vi "HAPS_PhaseGainSweep_Preamp_Chs.vi"() -> ()   [LabVIEW 2023, in "HAPS.lvlib"]
uses:
  HAPS.lvlib
  HAPS_SerialPort.ctl
  MCU_Function.ctl
  set_ele.ctl
  HAPS_MCU_ELE_Func.ctl
  R_S/R_S.lvlib
panel:
  in  "Init?":bool=TRUE
  in  "Gain sweep res":i32=3
  in  "Gain_Start":i32
  in  "Phase Sweep Step":i32=64
  in  "Gain Sweep Step":i32=13
  in  "comn_gain":i32=17
  out "Each_Phase_Sweep(sec)":dbl
  out "dup path":path
  out "Gain_step":i32
  out "channel":i32
  out "chain_id":i32
  out "group":i32
  out "array_id":i32
  in  "File_note":string
  out "Duration(sec)":dbl
  out "In-Phase : Phase(degree)":dbl[](graph)
  out "In-Phase : Gain(dB)":dbl[](graph)
  in  "Tx/Rx":enum16{"Rx", "Tx"}(ring)=enum."Tx"
  in  "array_id (MCU index)":i32
  in  "MCU_UART_addr":refnum<visa-resource-name>="COM8"
  in  "Target(degree)":dbl format="%#_13g"
  in  "SweepPoints":i32=11
  in  "sParameter":i32=21
  in  "Stop_Freq(GHz)":dbl=39.5
  in  "Start_Freq(GHz)":dbl=38.5
  in  "VISA resource name":refnum<visa-resource-name>="TCPIP0::192.168.119.45::inst0::INSTR"
  in  "HAPS_Equipment":enum16{"Keysight", "R&S"}(ring)=enum."R&S"
  # "HAPS_24x24_PhaseGain_Sweep_Preamp_v1.8"
  # "K:4718\nR:2798"
  # "VNA"
  # "Test Status"
  # "DUT"
  # "TCPIP0::192.168.1.31::hislip0::INSTR"
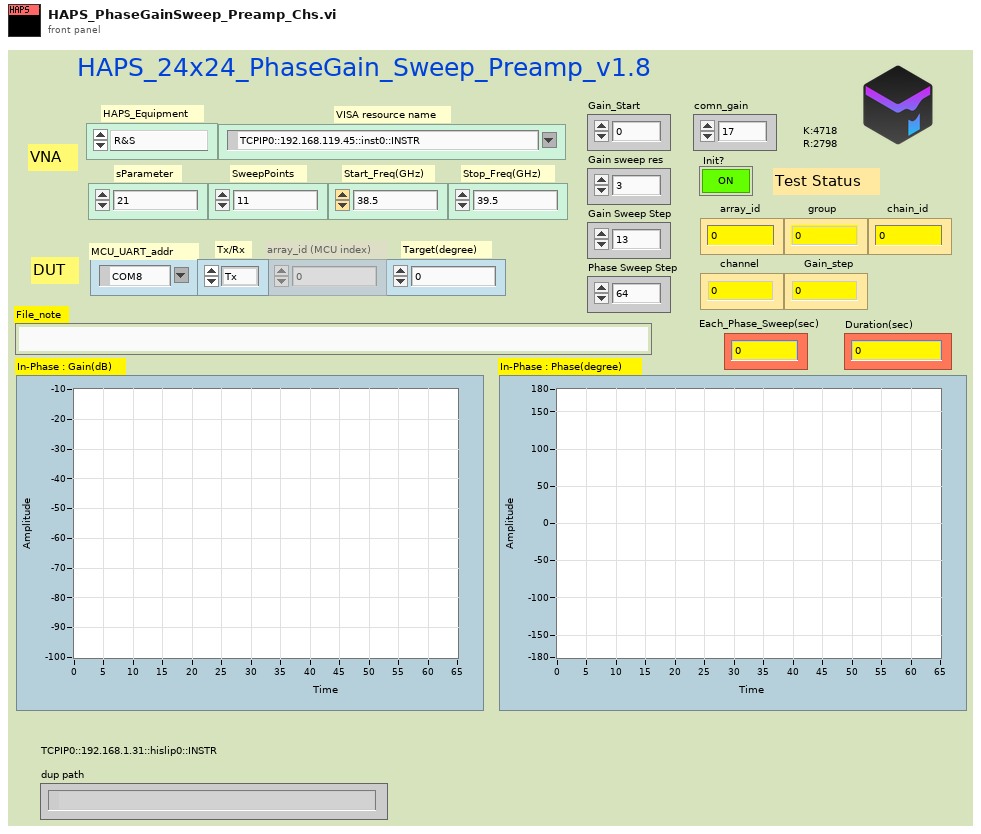
[diagram p1: front panel]
types:
  T1 = typedef "HAPS.lvlib/HAPS_SerialPort.ctl" = enum16{"Init", "Close", "CMD", "Flush"}
  T2 = typedef "HAPS.lvlib/HAPS_MCU_ELE_Func.ctl" = enum16{"array_init", "set_com_gain", "set_ch_gain_phase", "set_pd_range", "get_preamp_temp", "get_bfic_temp", "get_tx_pd", "ch_on", "ch_on_2", "ch_ctrl_all", "array_ctrl_src"}
  T3 = typedef "HAPS.lvlib/MCU_Function.ctl" = cluster{"Tx/Rx":enum16{"Rx", "Tx"}, "Enable?":enum16{"OFF", "On"}, "Source":enum16{"MCU", "ACU"}}
  T4 = typedef "HAPS.lvlib/set_ele.ctl" = cluster{"ch":i32, "chain_id":i32, "group":i32, "array_id":i32, "ele_phase":i32, "ele_gain":i32, "com_gain":i32, "pd_range":i32}
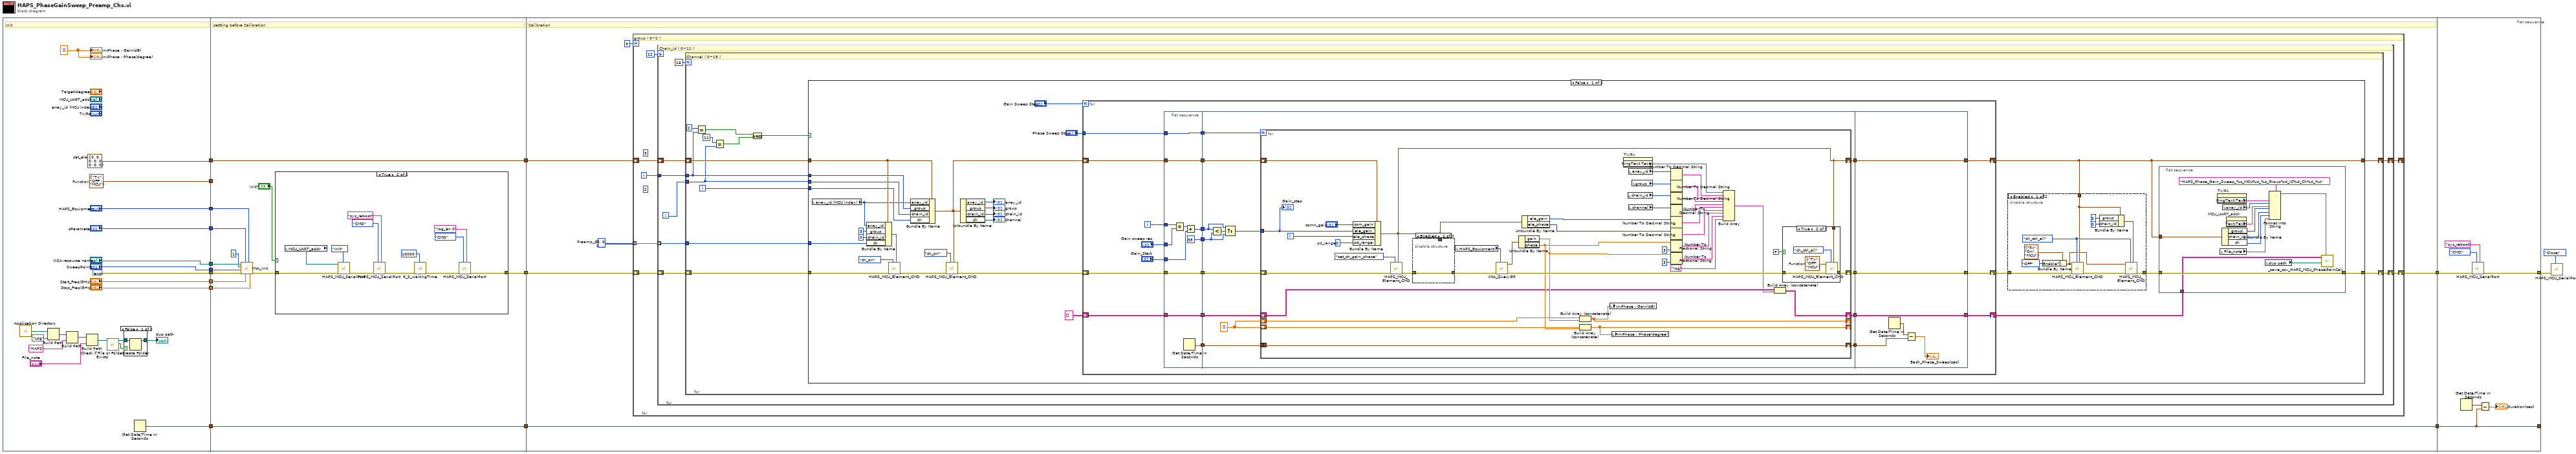
[diagram p0: block diagram]
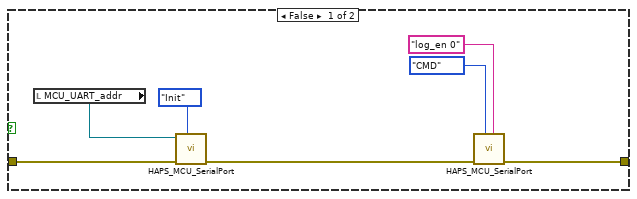
[diagram p3: hidden frame]
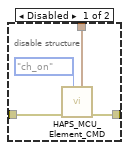
[diagram p4: hidden frame]
diagram:
  n1 = flat-sequence {
    tunnel: [w31] -> w17
    tunnel: [w38] -> w16
    tunnel: [errorcluster {"status"=FALSE, "code"=0, "source"=""} ("error in")] -> w14
    tunnel: ["sParameter"] -> w12
    tunnel: ["VISA resource name"] -> w11
    tunnel: ["Start_Freq(GHz)"] -> w10
    tunnel: ["Stop_Freq(GHz)"] -> w9
    tunnel: ["SweepPoints"] -> w8
    tunnel: ["HAPS_Equipment"] -> w7
    tunnel: [w28] -> w5
    tunnel: w17 -> [w54]
    tunnel: w16 -> [_]
    tunnel: [w54] -> w15
    tunnel: w14 -> [w53]
    tunnel: [w45] -> w13
    tunnel: w12 -> [w52]
    tunnel: w11 -> [w51]
    tunnel: w10 -> [w50]
    tunnel: w9 -> [w49]
    tunnel: w8 -> [w48]
    tunnel: w7 -> [w44]
    tunnel: [w43] -> w6
    tunnel: w5 -> [w43]
    tunnel: w15 -> [w78]
    tunnel: w13 -> [w79]
    tunnel: w6 -> [w76]
    tunnel: [w76] -> w4
    tunnel: [w74] -> w3
    tunnel: [w273] -> _
    tunnel: w4 -> [w273]
    tunnel: w3 -> [w269]
    tunnel: [w268] -> w2
    frame #0 {
      w29 = dbl[] []
      w31 = T4 {"ch"=0, "chain_id"=0, "group"=0, "array_id"=0, "ele_phase"=0, "ele_gain"=0, "com_gain"=0, "pd_range"=0}  # set_ele
      w38 = T3 {"Tx/Rx"=enum."Tx", "Enable?"=enum."OFF", "Source"=enum."MCU"}  # Function
      # "Init"
      n2 = call <vilib>:"Application Directory.vi"() -> ("Application Directory"=w26:path)
      n3 = Build Path(base path=w26, name or relative path="Log") -> (appended path=w27:path)
      n4 = Build Path(base path=w27, name or relative path="HAPS") -> (appended path=w23:path)
      n5 = Build Path(base path=w23, name or relative path="File_note") -> (appended path=w21:path)
      n6 = call <vilib>:"Check if File or Folder Exists.vi"("path"=w21) -> ("file or folder exists?"=w20:bool, "dup path"=w19:path)  [unwired: 8 in, 1 out]
      n7 = case shown="False" w20 {
        tunnel: w19 -> [w40 w41]
        tunnel: [w39 w41] -> w18
        frame False {
          n8 = Create Folder(path (use dialog)=w40) -> (created path=w39:path)  [unwired: 2 in, 2 out]
        }
        frame True {
        }
      }
      "dup path" <- w18
      n9 = Get Date/Time In Seconds() -> (seconds since 1Jan1904=w28:timestamp)
      "In-Phase : Gain(dB)" <- w29
      "In-Phase : Phase(degree)" <- w29
    }
    frame #1 {
      # "settting before Calibration"
      n10 = call "VNA_init.vi"("Stop_Freq(GHz)"=w49, "HAPS_MCU_CMD"=w44, "Start_Freq(GHz)"=w50, "sParameter"=w52, "error in"=w53, "SweepPoints"=w48, "Mark no."=1, "VISA resource name"=w51) -> ("error out"=w46:errorcluster)  [unwired: 3 in]
      n11 = case shown="True" "Init?" {
        tunnel: w46 -> [w58 w71]
        tunnel: [w55 w68] -> w45
        frame False {
          n12 = local read "MCU_UART_addr"() -> (w56:refnum<visa-resource-name>)
          n13 = call "HAPS_MCU_SerialPort.vi"("HAPS_SerialPort_Func"=HAPS_SerialPort."Init", "error in"=w58, "VISA resource name"=w56) -> ("error out"=w59:errorcluster)  [unwired: 6 in, 2 out]
          n14 = call "HAPS_MCU_SerialPort.vi"("Command"="log_en 0", "HAPS_SerialPort_Func"=enum16{"Init", "Close", "CMD"}."CMD" ("HAPS_SerialPort"), "error in"=w59) -> ("error out"=w55:errorcluster)  [unwired: 6 in, 2 out]
        }
        frame True {
          n15 = local read "MCU_UART_addr"() -> (w69:refnum<visa-resource-name>)
          n16 = call "HAPS_MCU_SerialPort.vi"("HAPS_SerialPort_Func"=HAPS_SerialPort."Init", "error in"=w71, "VISA resource name"=w69) -> ("error out"=w65:errorcluster)  [unwired: 6 in, 2 out]
          n17 = call "HAPS_MCU_SerialPort.vi"("Command"="sys_reboot", "HAPS_SerialPort_Func"=enum16{"Init", "Close", "CMD"}."CMD" ("HAPS_SerialPort"), "error in"=w65) -> ("error out"=w64:errorcluster)  [unwired: 6 in, 2 out]
          n18 = call "R_S_waitingTime.vi"("Waiting Time(ms)"=u32 10000, "error in"=w64) -> ("error out"=w63:errorcluster)  [unwired: 9 in]
          n19 = call "HAPS_MCU_SerialPort.vi"("Command"="log_en 0", "HAPS_SerialPort_Func"=enum16{"Init", "Close", "CMD"}."CMD" ("HAPS_SerialPort"), "error in"=w63) -> ("error out"=w68:errorcluster)  [unwired: 6 in, 2 out]
        }
      }
    }
    frame #2 {
      w75 = i32[][] [[2, 0, 0, 8, 8, 10, 11, 9, 9, 1, 1, 3], [3, 1, 1, 9, 9, 11, 13, 15, 15, 7, 7, 5], [5, 7, 7, 15, 15, 13, 14, 14, 6, 6, 4, 12]]  # Preamp_ch
      # "Calibration"
      n20 = for {
        N: 3 -> [_]
        shift-right: [w80] -> _
        shift-left: w78 -> [w84]
        shift-right: [w86] -> w74
        shift-left: w79 -> [w85]
        tunnel: w75 -> [w81] mode=indexing
        i -> [w82]
        (unwired) 2
        (unwired) 3
        # "group ( 0~2 )"
        n21 = for {
          N: 12 -> [_]
          shift-right: [w88] -> w80
          shift-left: w84 -> [w92]
          shift-right: [w87] -> w86
          shift-left: w85 -> [w93]
          tunnel: w82 -> [w91]
          tunnel: w81 -> [w89] mode=indexing
          i -> [w90]
          # "Chain_id ( 0~11 )"
          n22 = for {
            N: 16 -> [_]
            shift-right: [w104] -> w88
            shift-left: w92 -> [w107]
            shift-right: [w105] -> w87
            shift-left: w93 -> [w106]
            tunnel: w91 -> [w103]
            tunnel: w90 -> [w96]
            tunnel: w89 -> [w95]
            i -> [w97]
            # "Channel ( 0~15 )"
            n23 = Equal?(x=2, y=w103) -> (x = y?=w100:bool)
            n24 = Equal?(x=11, y=w96) -> (x = y?=w99:bool)
            n25 = And(x=w100, y=w99) -> (x .and. y?=w98:bool)
            n26 = case shown="False" w98 {
              tunnel: w107 -> [w125 w267]
              tunnel: w97 -> [w132 _]
              tunnel: w106 -> [w126 w266]
              tunnel: w103 -> [w134 _]
              tunnel: w96 -> [w133 _]
              tunnel: [w116 w266] -> w105
              tunnel: [w115 w267] -> w104
              tunnel: w95 -> [w120 _]
              frame False {
                n27 = local read "array_id (MCU index)"() -> (w123:i32)
                n28 = Bundle By Name(cluster=w125, "array_id"=w123, "group"=3, "chain_id"=0, "ch"=w120) -> (w124:T4)
                n29 = call "HAPS_MCU_Element_CMD.vi"("set_ele"=w124, "HAPS_MCU_ELE_Func."=HAPS_MCU_ELE_Func."ch_on", "error in"=w126) -> ("error out"=w127:errorcluster)  [unwired: 7 in, 1 out]
                n30 = Bundle By Name(cluster=w125, "array_id"=w123, "group"=w134, "chain_id"=w133, "ch"=w132) -> (w112:T4)
                n31 = call "HAPS_MCU_Element_CMD.vi"("set_ele"=w112, "HAPS_MCU_ELE_Func."=HAPS_MCU_ELE_Func."ch_on", "error in"=w127) -> ("error out"=w130:errorcluster)  [unwired: 7 in, 1 out]
                n32 = Unbundle By Name(w112) -> ("array_id"=→"array_id":i32, "group"=→"group":i32, "chain_id"=→"chain_id":i32, "ch"=→"channel":i32)
                n33 = for {
                  N: "Gain Sweep Step" -> [_]
                  shift-right: [w166] -> w129
                  shift-left: w130 -> [w167]
                  shift-right: [w165] -> w115
                  shift-left: w112 -> [w164]
                  shift-right: [w163] -> w114
                  shift-left: string[][] [] -> [w168]
                  tunnel: "Phase Sweep Step" -> [w152]
                  i -> [w162]
                  n34 = flat-sequence {
                    tunnel: w162 -> [w176]
                    tunnel: w164 -> [w177]
                    tunnel: w167 -> [w178]
                    tunnel: w168 -> [w179]
                    tunnel: [w179] -> w161
                    tunnel: [w178] -> w160
                    tunnel: [w177] -> w159
                    tunnel: [w175] -> w158
                    tunnel: [w174] -> w153
                    tunnel: w152 -> [w174]
                    tunnel: "Gain sweep res" -> [w173]
                    tunnel: "Gain_Start" -> [w171]
                    tunnel: [w170] -> w149
                    tunnel: [35 ("y")] -> w148
                    tunnel: w161 -> [w193]
                    tunnel: w160 -> [w192]
                    tunnel: w159 -> [w189]
                    tunnel: w158 -> [w186]
                    tunnel: [w191] -> w157
                    tunnel: [w190] -> w156
                    tunnel: [w188] -> w155
                    tunnel: [w185] -> w154
                    tunnel: w153 -> [w184]
                    tunnel: w149 -> [w182]
                    tunnel: w148 -> [w181]
                    tunnel: [w251] -> w163
                    tunnel: [w252] -> w165
                    tunnel: [w253] -> w166
                    tunnel: w157 -> [w253]
                    tunnel: w156 -> [w252]
                    tunnel: w155 -> [w251]
                    tunnel: w154 -> [w248]
                    frame #0 {
                      n35 = Multiply(x=w176, y=w173) -> (x*y=w172:i32)
                      n36 = Get Date/Time In Seconds() -> (seconds since 1Jan1904=w175:timestamp)
                      n37 = Add(x=w172, y=w171) -> (x+y=w170:i32)
                    }
                    frame #1 {
                      w187 = dbl[] []
                      n38 = Less?(x=w182, y=w181) -> (x < y?=w183:bool)
                      n39 = Select(t=w182, s=w183, f=w181) -> (s? t:f=w180:i32)
                      n40 = for {
                        N: w184 -> [_]
                        shift-right: [w217] -> _
                        shift-left: w187 -> [w219]
                        shift-right: [w216] -> _
                        shift-left: w187 -> [w218]
                        shift-right: [w214] -> w191
                        shift-left: w192 -> [w235]
                        shift-right: [w204] -> w190
                        shift-left: w189 -> [w236]
                        shift-right: [w208] -> w188
                        shift-left: w193 -> [w210]
                        tunnel: w180 -> [w196]
                        tunnel: w186 -> [w195]
                        shift-right: [w195] -> w185
                        shift-left: _ -> [_]
                        i -> [w194]
                        w233 = 0  # pd_range
                        n41 = Bundle By Name(cluster=w236, "com_gain"="comn_gain", "ele_gain"=w196, "ele_phase"=w194, "pd_range"=w233) -> (w204:T4)
                        n42 = call "HAPS_MCU_Element_CMD.vi"("set_ele"=w204, "HAPS_MCU_ELE_Func."=HAPS_MCU_ELE_Func."set_ch_gain_phase", "error in"=w235) -> ("error out"=w206:errorcluster)  [unwired: 7 in, 1 out]
                        n43 = disable-structure shown="Enabled" {
                          disable-tunnel: w206 -> [w240 w241]
                          disable-tunnel: [w239 w241] -> w205
                          disable-tunnel: w204 -> [w237 _]
                          frame Disabled {
                            n44 = call "HAPS_MCU_Element_CMD.vi"("set_ele"=w237, "HAPS_MCU_ELE_Func."=HAPS_MCU_ELE_Func."ch_on", "error in"=w240) -> ("error out"=w239:errorcluster)  [unwired: 7 in, 1 out]
                          }
                          frame Enabled {
                          }
                        }
                        n45 = local read "HAPS_Equipment"() -> (w221:enum16{"Keysight", "R&S"})
                        n46 = call "VNA_QueryGP.vi"("HAPS_Equipment"=w221, "error in"=w205) -> ("error out"=w215:errorcluster, "queryMarker"=w220:cluster{"gain":dbl, "phase":dbl})  [unwired: 8 in]
                        n47 = Unbundle By Name(w220) -> ("gain"=w211:dbl, "phase"=w212:dbl)
                        n48 = Unbundle By Name(w204) -> ("ele_gain"=w197:i32, "ele_phase"=w213:i32)
                        n49 = Build Array (concatenate)(w218, w212) -> (w216:dbl[])
                        n50 = Build Array (concatenate)(w219, w211) -> (w217:dbl[])
                        n51 = local write "In-Phase : Gain(dB)"(w217) -> ()
                        n52 = local write "In-Phase : Phase(degree)"(w216) -> ()
                        n53 = property on="Tx/Rx" class="Enum (strict)"() -> ("RingText.Text"=w198:string)  [unwired: 2 in, 2 out]
                        n54 = local read "chain_id"() -> (w223:i32)
                        n55 = local read "array_id"() -> (w225:i32)
                        n56 = local read "channel"() -> (w222:i32)
                        n57 = local read "group"() -> (w224:i32)
                        n58 = Number To Decimal String(number=w225) -> (decimal integer string=w199:string)  [unwired: 1 in]
                        n59 = Number To Decimal String(number=w224) -> (decimal integer string=w200:string)  [unwired: 1 in]
                        n60 = Number To Decimal String(number=w223) -> (decimal integer string=w201:string)  [unwired: 1 in]
                        n61 = Number To Decimal String(number=w222) -> (decimal integer string=w202:string)  [unwired: 1 in]
                        n62 = Number To Decimal String(number=w197) -> (decimal integer string=w203:string)  [unwired: 1 in]
                        n63 = Number To Decimal String(number=w213) -> (decimal integer string=w226:string)  [unwired: 1 in]
                        n64 = Number To Fractional String(number=w212, precision (6)=i16 3) -> (F-format string=w229:string)  [unwired: 2 in]
                        n65 = Number To Fractional String(number=w211, precision (6)=i16 3) -> (F-format string=w230:string)  [unwired: 2 in]
                        n66 = Build Array(w198, w199, w200, w201, w202, w203, w226, w229, w230, "log") -> (w209:string[])
                        n67 = Build Array (concatenate)(w210, w209) -> (w208:string[][])
                        n68 = case shown="True" FALSE {
                          tunnel: w215 -> [w242 w245]
                          tunnel: [w242 w244] -> w214
                          tunnel: w204 -> [_ w243]
                          frame False {
                          }
                          frame True {
                            w247 = T3 {"Tx/Rx"=enum."Tx", "Enable?"=enum."OFF", "Source"=enum."MCU"}  # Function
                            n69 = call "HAPS_MCU_Element_CMD.vi"("set_ele"=w243, "HAPS_MCU_ELE_Func."=HAPS_MCU_ELE_Func."ch_ctrl_all", "error in"=w245, "Function"=w247) -> ("error out"=w244:errorcluster)  [unwired: 6 in, 1 out]
                          }
                        }
                        "Gain_step" <- w196
                      }
                    }
                    frame #2 {
                      n70 = Get Date/Time In Seconds() -> (seconds since 1Jan1904=w249:timestamp)
                      n71 = Subtract(x=w249, y=w248) -> (x-y=→"Each_Phase_Sweep(sec)":dbl)
                    }
                  }
                }
                n72 = disable-structure shown="Enabled" {
                  disable-tunnel: w129 -> [w264 w265]
                  disable-tunnel: [w260 w265] -> w117
                  disable-tunnel: w115 -> [w255 _]
                  frame Enabled {
                    w259 = HAPS_MCU_ELE_Func."ch_ctrl_all" ("HAPS_MCU_ELE_Func.")
                    n73 = Bundle By Name(cluster=T3 {"Tx/Rx"=enum."Rx", "Enable?"=enum."On", "Source"=enum."MCU"} ("Function"), "Enable?"=enum16{"OFF", "On"}."OFF") -> (w258:T3)
                    n74 = call "HAPS_MCU_Element_CMD.vi"("set_ele"=w255, "HAPS_MCU_ELE_Func."=w259, "error in"=w264, "Function"=w258) -> ("error out"=w261:errorcluster)  [unwired: 6 in, 1 out]
                    n75 = Bundle By Name(cluster=w255, "group"=3, "chain_id"=0) -> (w254:T4)
                    n76 = call "HAPS_MCU_Element_CMD.vi"("set_ele"=w254, "HAPS_MCU_ELE_Func."=w259, "error in"=w261, "Function"=w258) -> ("error out"=w260:errorcluster)  [unwired: 6 in, 1 out]
                  }
                  frame Disabled {
                  }
                }
                n77 = flat-sequence {
                  tunnel: w115 -> [w141]
                  tunnel: w117 -> [w138]
                  tunnel: [w138] -> w116
                  tunnel: w114 -> [w135]
                  frame #0 {
                    n78 = property on="Tx/Rx" class="Enum (strict)"() -> ("RingText.Text"=w145:string)  [unwired: 2 in, 2 out]
                    n79 = local read "File_note"() -> (w136:string)
                    n80 = Unbundle By Name(w141) -> ("group"=w143:i32, "chain_id"=w140:i32, "ch"=w137:i32)
                    n81 = local read "array_id"() -> (w144:i32)
                    n82 = property on="MCU_UART_addr" class="VISAName"() -> ("Text.Text"=w147:string)  [unwired: 2 in, 2 out]
                    n83 = local read "dup path"() -> (w139:path)
                    n84 = Format Into String(format string="HAPS_Phase_Gain_Sweep_%s_MCU%d_%s_Group%d_IC%d_Ch%d_%s", w145, w144, w147, w143, w140, w137, w136) -> (resulting string=w146:string)  [unwired: 2 in, 1 out]
                    n85 = call "_save_csv_HAPS_MCU_PhaseGainCali.vi"("NoteName"=w146, "dup path"=w139, "array in"=w135) -> ()  [unwired: 8 in, 1 out]
                  }
                }
              }
              frame True {
              }
            }
          }
        }
      }
    }
    frame #3 {
      n86 = Get Date/Time In Seconds() -> (seconds since 1Jan1904=w274:timestamp)
      n87 = call "HAPS_MCU_SerialPort.vi"("Command"="sys_reboot", "HAPS_SerialPort_Func"=enum16{"Init", "Close", "CMD"}."CMD" ("HAPS_SerialPort"), "error in"=w269) -> ("error out"=w268:errorcluster)  [unwired: 6 in, 2 out]
      n88 = Subtract(x=w274, y=w273) -> (x-y=→"Duration(sec)":dbl)
    }
  }
  n89 = call "HAPS_MCU_SerialPort.vi"("HAPS_SerialPort_Func"=HAPS_SerialPort."Close", "error in"=w2) -> ()  [unwired: 7 in, 3 out]
